vi "Read Optimisation Strategy from string.vi"(0 "String":string) -> (1 "Optimisation Strategy":T1, 2 "value":dbl)   [LabVIEW 2020, in "TALOS.lvlib" / "Run Utilities.lvlib" / "Optimiser Cell.lvclass"]
uses:
  Optimiser Cell.lvclass
  Optimisation Strategy.ctl
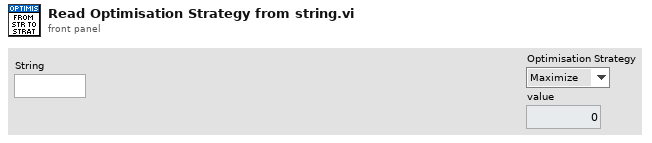
[diagram p1: front panel]
types:
  T1 = typedef "TALOS.lvlib/Run Utilities.lvlib/Optimiser Cell.lvclass/Optimisation Strategy.ctl" = enum16{"Maximize", "Minimize", "Value"}
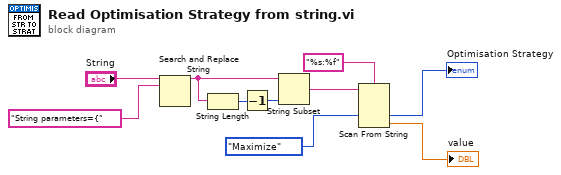
[diagram p0: block diagram]
diagram:
  n1 = Search and Replace String(input string="String", search string="String parameters={") -> (result string=w7:string)  [unwired: 6 in, 3 out]
  n2 = String Length(string=w7) -> (length=w6:i32)
  n3 = Decrement(x=w6) -> (x-1=w5:i32)
  n4 = String Subset(string=w7, length (rest)=w5) -> (substring=w4:string)  [unwired: 1 in]
  n5 = Scan From String(format string="%s:%f", input string=w4, default 1=Optimisation_Strategy."Maximize" ("Optimisation Strategy")) -> (output 1=→"Optimisation Strategy":T1, output 2=→"value":dbl)  [unwired: 3 in, 3 out]
